vi "RD Analog In Configure.vi"(8 "error in (no error)":errorcluster caption="错误输入（无错误）", 10 "run":bool, 11 "handle":u64) -> (0 "error out":errorcluster caption="错误输出", 2 "function return":i32, 3 "handle out":u64)   [LabVIEW 2018, in "InstrumentsPlayground.lvlib"]
doc: "CLIFFAPI int CliffAnalogInConfigure(FT_HANDLE handle,bool run);\nrun: 1 for start once in manule trigger mode; infinite for none or auto trigger mode."
uses:
  InstrumentsPlayground.lvlib
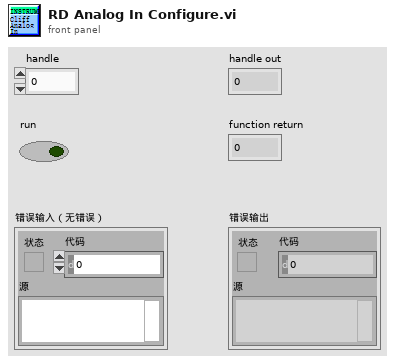
[diagram p1: front panel]
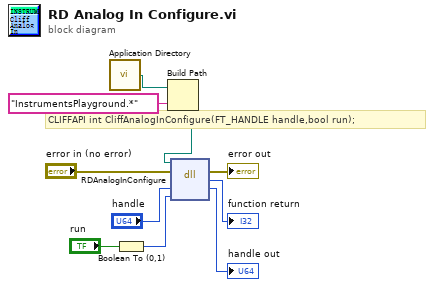
[diagram p0: block diagram]
diagram:
  # "CLIFFAPI int CliffAnalogInConfigure(FT_HANDLE handle,bool run);"
  n1 = call <vilib>:"Application Directory.vi"() -> ("Application Directory"=w2:path)
  n2 = Boolean To (0,1)(Boolean="run") -> (0, 1=w6:i16)
  n3 = Build Path(base path=w2, name or relative path="InstrumentsPlayground.*" ("名称或相对路径")) -> (appended path=w1:path)
  n4 = dll-call lib="E:/work/YZCourse_Xtext/Cliff/API/LabVIEW lib/InstrumentsPlayground.*" fn="RDAnalogInConfigure"(path in=w1, error in="error in (no error)", "handle"="handle", "run"=w6) -> (error out=→"error out":errorcluster, "返回类型"=→"function return":i32, "handle"=→"handle out":u64)  [unwired: 2 in, 1 out]
